vi "handler tester.vi"() -> ()   [LabVIEW 2021]
uses:
  TCP states.ctl
panel:
  out "Response":string
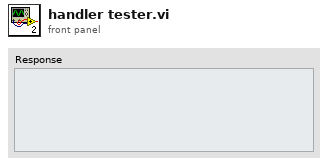
[diagram p1: front panel]
types:
  T1 = typedef "TCP states.ctl" = string
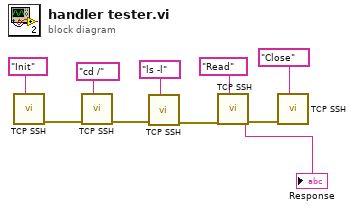
[diagram p0: block diagram]
diagram:
  n1 = call "TCP SSH.vi"("States"=T1 "Init") -> ("Error  Out"=w6:errorcluster)  [unwired: 8 in, 1 out]
  n2 = call "TCP SSH.vi"("States"=T1 "cd /", "Error In"=w6) -> ("Error  Out"=w2:errorcluster)  [unwired: 7 in, 1 out]
  n3 = call "TCP SSH.vi"("States"=T1 "ls -l", "Error In"=w2) -> ("Error  Out"=w1:errorcluster)  [unwired: 7 in, 1 out]
  n4 = call "TCP SSH.vi"("States"=T1 "Read", "Error In"=w1) -> ("Error  Out"=w5:errorcluster, "Response"=→"Response":string)  [unwired: 7 in]
  n5 = call "TCP SSH.vi"("States"=T1 "Close", "Error In"=w5) -> ()  [unwired: 7 in, 2 out]
